vi "Write Zone.vi"(8 "error in (no error)":errorcluster, 10 "Zone.lvclass":refnum<class "Zone.lvclass">, 11 "Role_v2 in":refnum<class "Role_v2.lvclass">) -> (0 "error out":errorcluster, 3 "Role_v2 out":refnum<class "Role_v2.lvclass">)   [LabVIEW 2023]
uses:
  Role_v2.lvclass
  Zone_class/Zone.lvclass
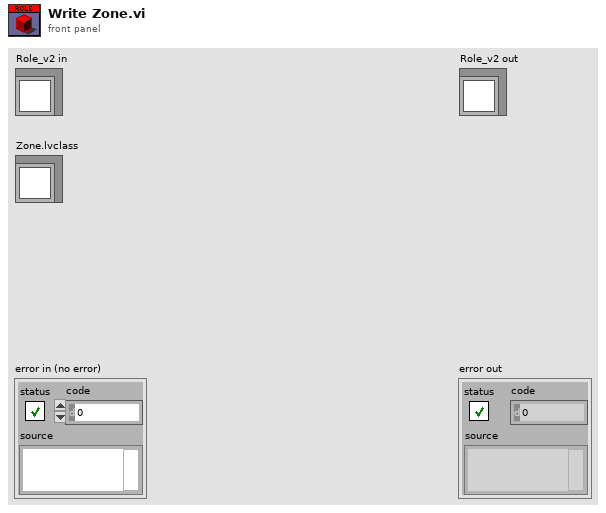
[diagram p1: front panel]
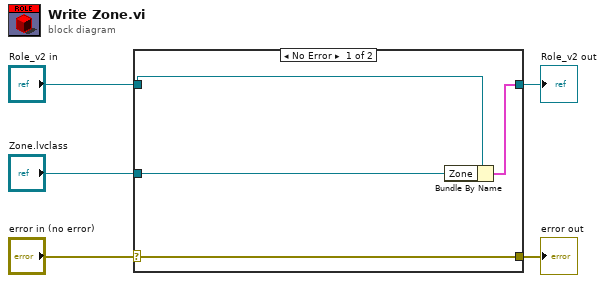
[diagram p0: block diagram]
diagram:
  n1 = case shown="No Error" "error in (no error)" {
    selector: "error in (no error)" -> [w9 w10]
    tunnel: [w9 w10] -> w4
    tunnel: [w7 w11] -> w2
    tunnel: "Role_v2 in" -> [w8 w11]
    tunnel: "Zone.lvclass" -> [w6 _]
    frame No Error {
      n2 = Bundle By Name(cluster=w8, "Zone"=w6) -> (w7:cluster{})
    }
    frame Error {
    }
  }
  "error out" <- w4
  "Role_v2 out" <- w2
